vi "Read Connection String.vi"(8 "error in (no error)":errorcluster, 11 "Interface in":refnum<class "Interface.lvclass">) -> (0 "error out":errorcluster, 2 "Connection String":string, 3 "Interface out":refnum<class "Interface.lvclass">)   [LabVIEW 2016, in "Configuration.lvlib" / "Interface.lvclass"]
doc: "Read connection string from class private data."
uses:
  Interface.lvclass
  Interface.lvclass/Interface.ctl
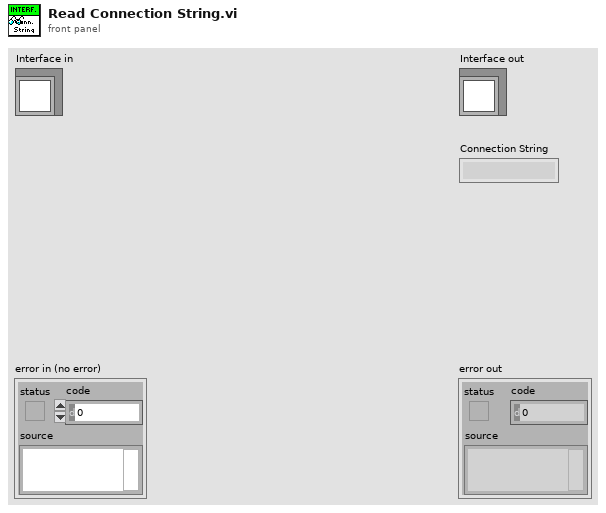
[diagram p1: front panel]
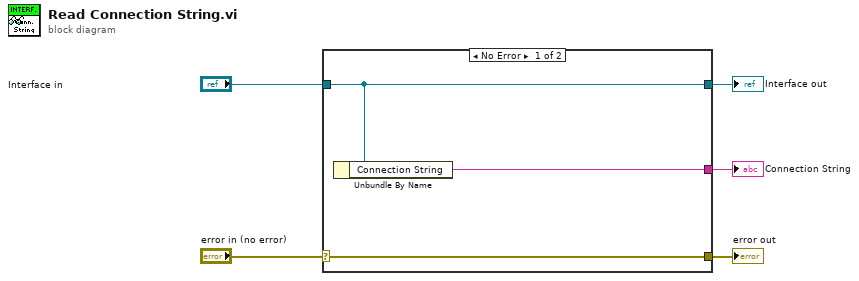
[diagram p0: block diagram]
diagram:
  n1 = case shown="No Error" "error in (no error)" {
    selector: "error in (no error)" -> [w8 w9]
    tunnel: [w8 w9] -> w4
    tunnel: [w7 w10] -> w2
    tunnel: "Interface in" -> [w7 w10]
    tunnel: [w6 _] -> w1
    frame No Error {
      n2 = Unbundle By Name(w7) -> ("Connection String"=w6:string)
    }
    frame Error {
    }
  }
  "error out" <- w4
  "Interface out" <- w2
  "Connection String" <- w1
